vi "PXIe-433x Initialization VI.vi"(8 "error in (no error)":errorcluster, 10 "Custom XML":string, 11 "Device Item Ref in":T1 format="%.0x") -> (0 "error out":errorcluster, 3 "Device Item Ref out":T1 format="%.0x")   [LabVIEW 2010, in "PXIe-433x Custom Device.lvlib"]
uses:
  PXIe-433x Custom Device.lvlib
  <vilib>/NI VeriStand/Custom Device API/Custom Device Item Ref.ctl
  <vilib>/NI VeriStand/Custom Device API/Custom Device Channel.ctl
  <vilib>/NI VeriStand/Custom Device API/Custom Device Channel Type.ctl
  <vilib>/NI Veristand/Custom Device API/Custom Device Loop Type.ctl
  Global.vi
  <vilib>/NI Veristand/Custom Device API/Custom Device API.lvlib
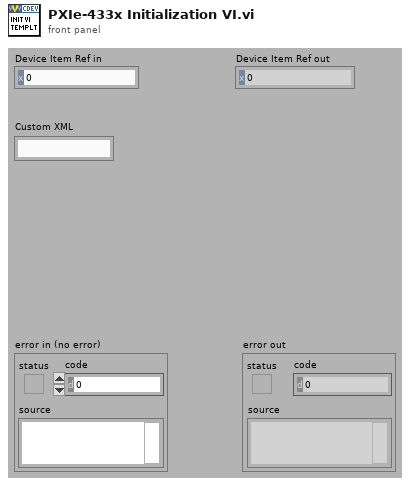
[diagram p1: front panel]
types:
  T1 = typedef "Custom Device API.lvlib/Custom Device Item Ref.ctl" = u64
  T2 = typedef "Custom Device API.lvlib/Custom Device Channel.ctl" = cluster{"Type":T3, "Units":string, "Default Value":dbl, "Faultable":bool, "Scalable":bool}
  T3 = typedef "Custom Device API.lvlib/Custom Device Channel Type.ctl" = enum16{"Input", "Output"}
  T4 = typedef "Custom Device API.lvlib/Custom Device Loop Type.ctl" = enum32{"While Loop", "Timed Loop"}
  T5 = typedef "PXIe-433x Custom Device.lvlib/Max Value.ctl" = dbl
  T6 = typedef "PXIe-433x Custom Device.lvlib/Sensor Type.ctl" = enum16{"Strain", "Force", "Pressure", "Torque"}
  T7 = typedef "PXIe-433x Custom Device.lvlib/Min Value.ctl" = dbl
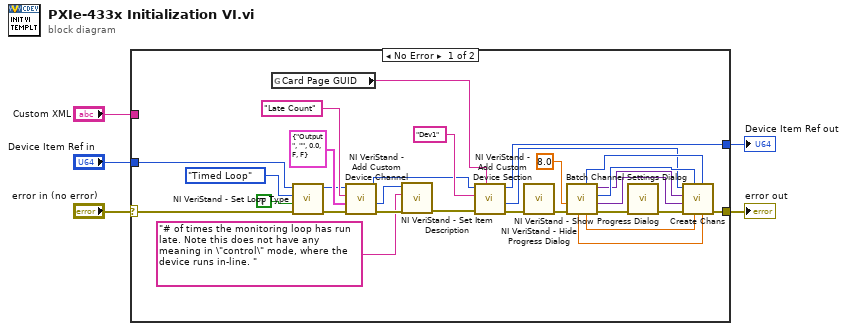
[diagram p0: block diagram]
diagram:
  n1 = case shown="No Error" "error in (no error)" {
    selector: "error in (no error)" -> [w6 w36]
    tunnel: [w27 w36] -> w5
    tunnel: [w16 w35] -> w3
    tunnel: "Device Item Ref in" -> [w23 w35]
    tunnel: "Custom XML" -> [_ _]
    frame No Error {
      n2 = global read "Global.vi" "Card Page GUID"() -> (w18:string)
      n3 = call <vilib>:"NI VeriStand - Set Loop Type.vi"("error in (no error)"=w6, "Use Device Clock (Timed Loops only)"=TRUE, "Loop type"=Custom_Device_Loop_Type."Timed Loop", "Device Ref in"=w23) -> ("error out"=w15:errorcluster, "Device Ref out"=w14:T1)  [unwired: 6 in]
      n4 = call <vilib>:"NI VeriStand - Add Custom Device Channel.vi"("error in (no error)"=w15, "Channel"=T2 {"Type"=enum."Output", "Units"="", "Default Value"=0.0, "Faultable"=FALSE, "Scalable"=FALSE}, "Channel Name"="Late Count", "Parent Ref in"=w14) -> ("error out"=w11:errorcluster, "Channel Ref"=w8:T1, "Parent Ref out"=w7:T1)  [unwired: 4 in, 1 out]
      n5 = call <vilib>:"NI VeriStand - Set Item Description.vi"("error in (no error)"=w11, "Description"="# of times the monitoring loop has run late. Note this does not have any meaning in \"control\" mode, where the device runs in-line. ", "Item Ref in"=w8) -> ("error out"=w10:errorcluster)  [unwired: 6 in, 2 out]
      n6 = call <vilib>:"NI VeriStand - Add Custom Device Section.vi"("GUID (Default Section)"=w18, "error in (no error)"=w10, "Section Name"="Dev1", "Parent Ref in"=w7) -> ("error out"=w13:errorcluster, "Section Ptr"=w12:T1, "Parent Ref out"=w16:T1)  [unwired: 4 in, 1 out]
      n7 = call <vilib>:"NI VeriStand - Hide Progress Dialog.vi"("error in (no error)"=w13) -> ("error out"=w28:errorcluster)  [unwired: 10 in]
      n8 = call "Batch Channel Settings Dialog.vi"("error in (no error)"=w28, "Data Entry Limits:Maximum"=8.0) -> ("error out"=w34:errorcluster, "scaling information"=w25:variant, "# of Chans"=w31:u8, "bridge information"=w26:variant, "Maximum Value"=w30:T5, "Sensor Type"=w24:T6, "Minimum Value"=w29:T7)  [unwired: 3 in]
      n9 = call <vilib>:"NI VeriStand - Show Progress Dialog.vi"("error in (no error)"=w34) -> ("error out"=w33:errorcluster)  [unwired: 10 in]
      n10 = call "Create Chans.vi"("Minimum Value"=w29, "Sensor Type"=w24, "Maximum Value"=w30, "# of Chans"=w31, "error in"=w33, "scaling information"=w25, "bridge information"=w26, "Item Ref in"=w12) -> ("error out"=w27:errorcluster)  [unwired: 2 in, 1 out]
    }
    frame Error {
    }
  }
  "error out" <- w5
  "Device Item Ref out" <- w3
